vi "initialize.vi"(0 "14bits":bool=TRUE) -> (3 "session out":refnum<k35>, 4 "available cameras":cluster{string[], string[]}, 6 "error out":errorcluster)   [LabVIEW 2022 SP3]
uses:
  Program Files/National Instruments/LabVIEW 2022/examples/Connectivity/Python/support/PythonVersionsEnum.ctl
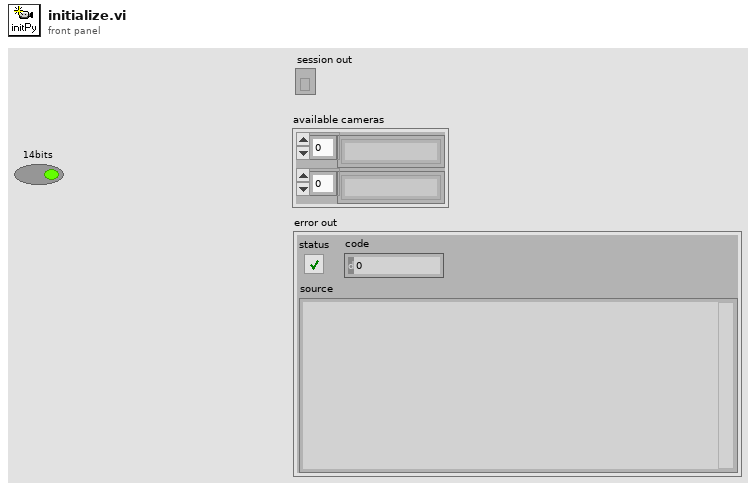
[diagram p1: front panel]
types:
  T1 = typedef "PythonVersionsEnum.ctl" = enum16{"3.6", "3.7", "3.8", "3.9"}
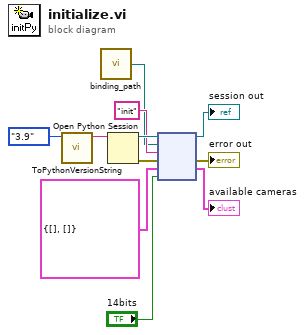
[diagram p0: block diagram]
diagram:
  n1 = call "ToPythonVersionString.vi"("python version"=PythonVersionsEnum."3.9") -> ("python version string"=w10:string)  [unwired: 10 in]
  n2 = call "binding_path.vi"() -> ("appended path"=w1:path)
  n3 = Open Python Session(python version=w10) -> (session out=w9:refnum<k35>, error out=w8:errorcluster)  [unwired: 2 in]
  n4 = node(w9, w1, "init" ("function name"), w8, cluster{string[], string[]} {[], []}, "14bits") -> (→"session out":refnum<k35>, →"error out":errorcluster, →"available cameras":cluster{string[], string[]})  [unwired: 1 in, 2 out]
